vi "ReadWrite.Data.Read.vi"(7 "Ignore Reset Values?":bool=TRUE, 8 "error in":errorcluster, 10 "timeout ms":i32, 11 "Ref":T1) -> (0 "error out":errorcluster, 1 "Timeout?":bool, 2 "Data":dbl[](array[numeric]), 3 "Detect?":bool[](array[boolean]))   [LabVIEW 2024, in "VS Plugin Data Access Engine.lvlib" / "Plugin Data Access Engine.lvclass"]
uses:
  Plugin Data Access Engine.lvclass
  Types/ReadWrite.DVR.ctl
  Access Type Classes/ReadWrite/ReadWrite.lvclass
  Plugin Data Access Engine.lvclass/Plugin Data Access Engine.ctl
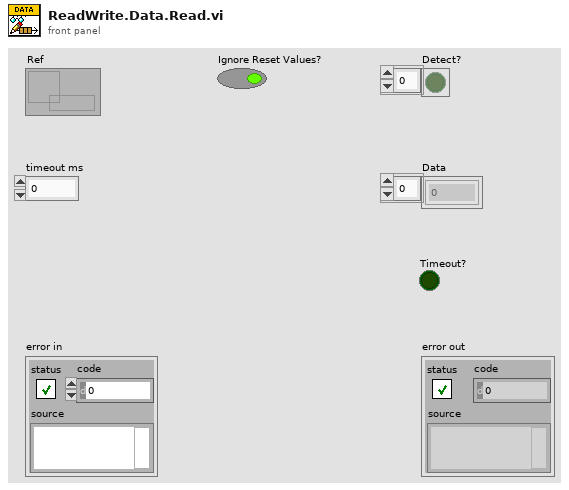
[diagram p1: front panel]
types:
  T1 = typedef "VS Plugin Data Access Engine.lvlib/Plugin Data Access Engine.lvclass/ReadWrite.DVR.ctl" = refnum<data-value>
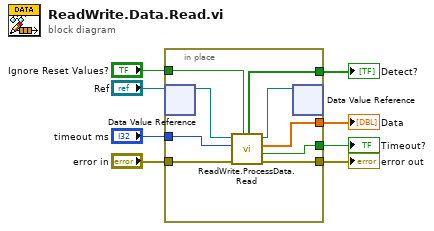
[diagram p0: block diagram]
diagram:
  n1 = in-place {
    in-place-border: "error in" -> [w17]
    in-place-border: [w16] -> w7
    in-place-border: "timeout ms" -> [w14]
    in-place-border: [w12] -> w4
    in-place-border: [w11] -> w3
    in-place-border: [w10] -> w2
    in-place-border: "Ignore Reset Values?" -> [w9]
    n2 = in-place-dvr #1("Ref") -> (w15:refnum<class "ReadWrite.lvclass">)  [unwired: 1 out]
    n3 = call "ReadWrite.ProcessData.Read.vi"("Ignore Reset Values?"=w9, "error in"=w17, "timeout ms"=w14, "ReadWrite in"=w15) -> ("error out"=w16:errorcluster, "Timeout?"=w11:bool, "Values"=w12:dbl[], "ReadWrite out"=w13:refnum<class "ReadWrite.lvclass">, "Detect?"=w10:bool[])  [unwired: 3 in]
    n4 = in-place-dvr #1(w13) -> ()  [unwired: 2 out]
  }
  "error out" <- w7
  "Data" <- w4
  "Timeout?" <- w3
  "Detect?" <- w2
